vi "line to strings with terminal type.vi"(11 "line":T1) -> (3 "strings":string[](array[string]))   [LabVIEW 2015, in "io editor node.lvclass"]
uses:
  io editor node.lvclass
  table line.ctl
  <vilib>/NI/Tag Bus Module Framework/channel/TBM channel.lvclass
  fpga channel/fpga channel.lvclass
  <vilib>/NI/Tag Bus/tag/tag descriptor.lvclass/tag descriptor.ctl
  <vilib>/NI/Tag Bus Module Framework/channel/TBM channel.lvclass/TBM channel.ctl
  fpga channel/fpga channel.lvclass/fpga channel.ctl
  fpga channel/Read FXP type.vi
  <vilib>/NI/Tag Bus/tag/read tag name.vi
  <vilib>/NI/Tag Bus Module Framework/channel/Read channel classification.vi
  <vilib>/NI/Tag Bus/tag/read data type.vi
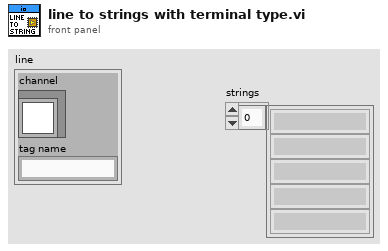
[diagram p1: front panel]
types:
  T1 = typedef "io editor node.lvclass/table line.ctl" = cluster{"channel":refnum<class "TBM channel.lvclass">, "tag name":string}
  T2 = typedef "TBM channel.lvclass/channel classification.ctl" = enum16{"input data", "output data", "processing parameter", "processing result"}
  T3 = typedef "tag bus.lvlib/tag descriptor.lvclass/Data Type.ctl" = enum16{"Double", "Single", "I64", "I32", "I16", "I8", "U64", "U32", "U16", "U8", "Boolean", "String", "Array of Double", "Array of Single", "Array of I64", "Array of I32", "Array of I16", "Array of I8", "Array of U64", "Array of U32", "Array of U16", "Array of U8", "Array of Boolean", "Array of String"}
  T4 = typedef "LVFixedPointRepBitsTypeDef.ctl" = cluster{"Signed":bool, "Word Length":u32, "Integer Word Length":i32}
  T5 = typedef "io editor node.lvclass/permissions.ctl" = enum32{"Read from Indicator", "Write to Control"}
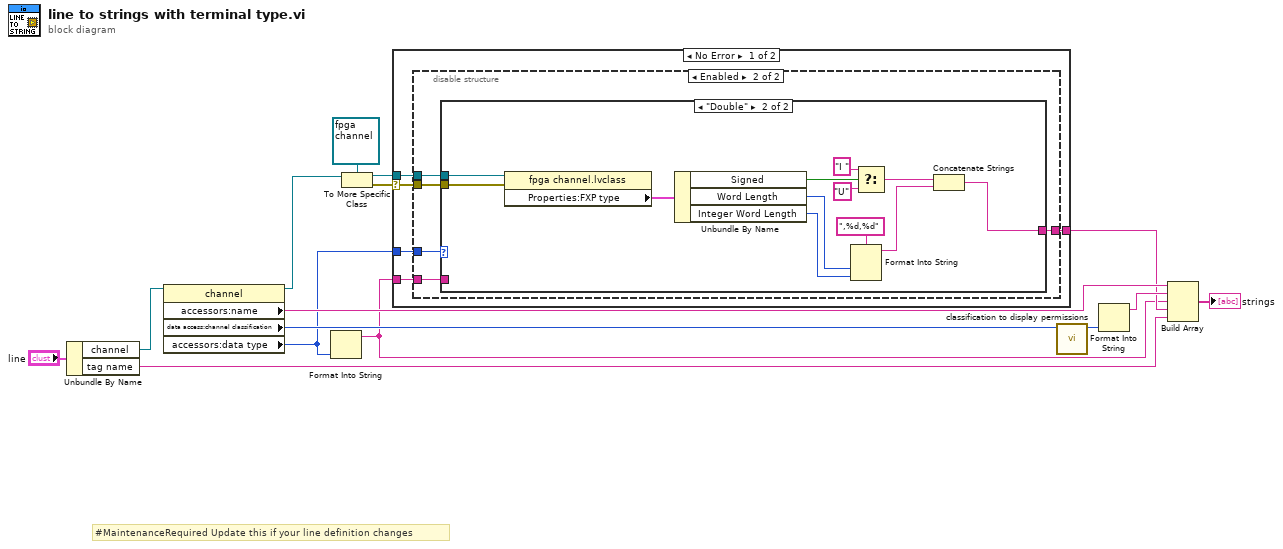
[diagram p0: block diagram]
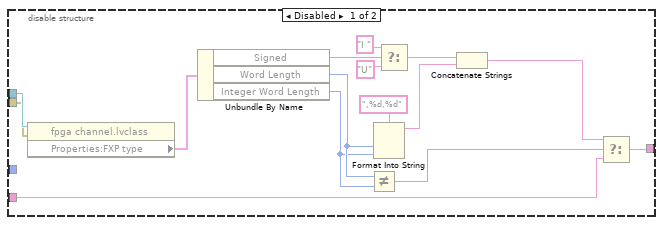
[diagram p2: hidden frame]
diagram:
  # "#MaintenanceRequired Update this if your line definition changes"
  n1 = Unbundle By Name("line") -> ("channel"=w11:refnum<class "TBM channel.lvclass">, "tag name"=w5:string)
  n2 = property class="channel"(reference=w11) -> (reference out=w8:refnum<class "TBM channel.lvclass">, "accessors:name"=w9:string, "data access:channel classification"=w10:T2, "accessors:data type"=w1:T3)  [unwired: 1 in, 1 out]
  n3 = Format Into String(w1) -> (resulting string=w3:string)  [unwired: 3 in, 1 out]
  n4 = To More Specific Class(target class=refnum<class "fpga channel.lvclass"> refnum ("fpga channel.lvclass"), reference=w8) -> (specific class reference=w6:refnum<class "fpga channel.lvclass">, error out=w7:errorcluster)  [unwired: 1 in]
  n5 = case shown="No Error" w7 {
    selector: w7 -> [w18 _]
    tunnel: w6 -> [w20 _]
    tunnel: [w19 w54] -> w4
    tunnel: w3 -> [w17 w54]
    tunnel: w1 -> [w16 _]
    frame No Error {
      n6 = disable-structure shown="Enabled" {
        disable-tunnel: w20 -> [w35 w40]
        disable-tunnel: [w34 w39] -> w19
        disable-tunnel: w18 -> [w33 w38]
        disable-tunnel: w17 -> [w32 w37]
        disable-tunnel: w16 -> [_ w36]
        frame Disabled {
          n7 = property class="fpga channel.lvclass"(reference=w35, error in=w33) -> ("Properties:FXP type"=w31:T4)  [unwired: 2 out]
          n8 = Unbundle By Name(w31) -> ("Signed"=w25:bool, "Word Length"=w24:u32, "Integer Word Length"=w23:i32)
          n9 = Not Equal?(x=w24, y=w23) -> (x != y?=w22:bool)
          n10 = Format Into String(format string=",%d,%d", w24, w23) -> (resulting string=w29:string)  [unwired: 2 in, 1 out]
          n11 = Select(t="I " ("string"), s=w25, f="U") -> (s? t:f=w28:string)
          n12 = Concatenate Strings(w28, w29) -> (w21:string)
          n13 = Select(t=w21, s=w22, f=w32) -> (s? t:f=w34:string)
        }
        frame Enabled {
          n14 = case shown="\"Double\"" w36 {
            tunnel: w40 -> [_ w53]
            tunnel: [w41 w42] -> w39
            tunnel: w38 -> [_ w52]
            tunnel: w37 -> [w41 _]
            frame Default {
            }
            frame "Double" {
              n15 = property class="fpga channel.lvclass"(reference=w53, error in=w52) -> ("Properties:FXP type"=w51:T4)  [unwired: 2 out]
              n16 = Unbundle By Name(w51) -> ("Signed"=w45:bool, "Word Length"=w44:u32, "Integer Word Length"=w43:i32)
              n17 = Format Into String(format string=",%d,%d", w44, w43) -> (resulting string=w49:string)  [unwired: 2 in, 1 out]
              n18 = Select(t="I " ("string"), s=w45, f="U") -> (s? t:f=w48:string)
              n19 = Concatenate Strings(w48, w49) -> (w42:string)
            }
          }
        }
      }
    }
    frame Error {
    }
  }
  n20 = call "classification to display permissions.vi"("channel classification"=w10) -> ("permissions"=w13:T5)  [unwired: 10 in]
  n21 = Format Into String(w13) -> (resulting string=w12:string)  [unwired: 3 in, 1 out]
  n22 = Build Array(w9, w12, w3, w4, w5) -> (→"strings":string[])
